vi "subExportDependencyItemRuleContent.vi"(8 "error in (no error)":errorcluster, 9 "Expand?":bool, 11 "IDependencyItemRule in":refnum<class "IDependencyItemRule.lvclass">) -> (0 "error out":errorcluster, 1 "Links":T1, 2 "Nodes":T1, 3 "IDependencyItemRule out":refnum<class "IDependencyItemRule.lvclass">)   [LabVIEW 2020, in "DefaultExtensions.lvlib" / "CGrapherDGML.lvclass"]
uses:
  CGrapherDGML.lvclass
  obj/Addons/LabVIEWObjectInterfaces.lvlibp/LabVIEWObjectInterfaces/IDependencyItemRule/IDependencyItemRule.lvclass
  C:/DependencyInspector/obj/Addons/LabVIEWObjectInterfaces.lvlibp/LabVIEWObjectInterfaces/ILabVIEWItem/ILabVIEWItem.lvclass
  obj/Addons/LabVIEWItem.lvlibp/LabVIEWItem/CLabVIEWItem/ConnectionSet.ctl
  84b6f64b-e02b-4565-8a95-97306d3fff3e.vi
  5ae37459-432d-44eb-8d2b-a2ae9b2d80af.vi
  0dec89c7-531e-457a-9eb0-0c91c63ee5dd.vi
  obj/Addons/LabVIEWItem.lvlibp/LabVIEWItem/CLabVIEWItem/CLabVIEWItem.lvclass
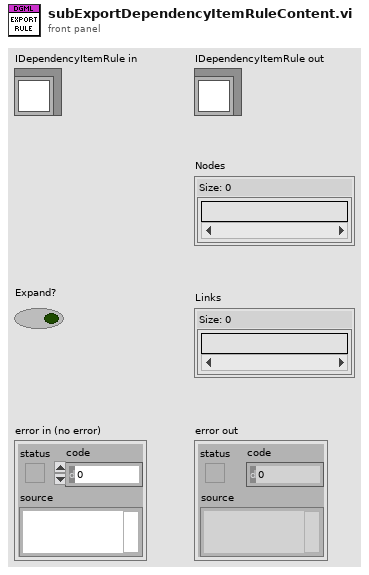
[diagram p1: front panel]
types:
  T1 = typedef "LabVIEWItem.lvlibp/CLabVIEWItem.lvclass/ConnectionSet.ctl" = set{string}
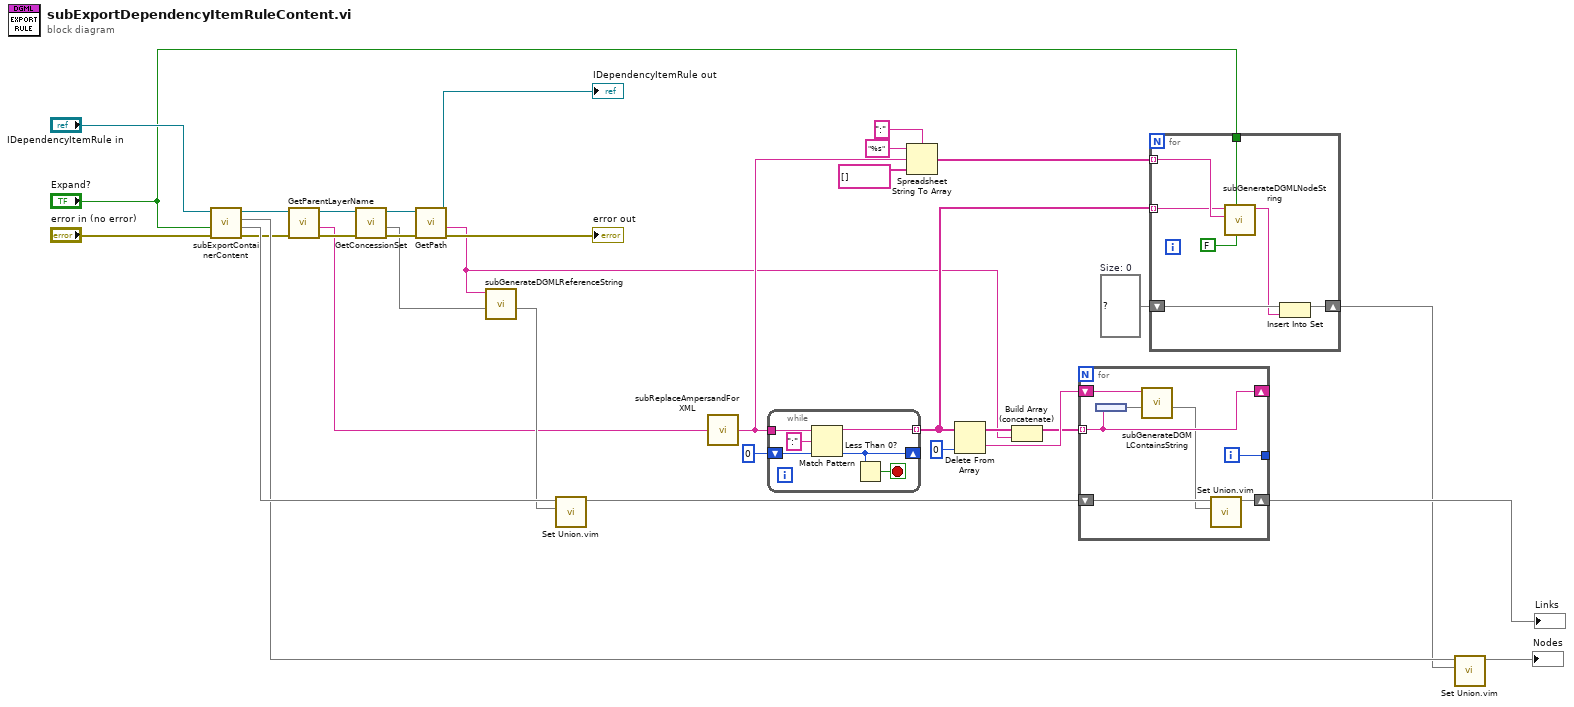
[diagram p0: block diagram]
diagram:
  w19 = set{string} {}  # Size: 0
  n1 = call "subExportContainerContent.vi"("error in (no error)"="error in (no error)", "Expand?"="Expand?", "ILabVIEWItem in"="IDependencyItemRule in") -> ("error out"=w4:errorcluster, "Links"=w30:T1, "Nodes"=w18:T1, "ILabVIEWItem out"=w5:refnum<class "IDependencyItemRule.lvclass">)  [unwired: 5 in]
  n2 = call-dynamic "GetParentLayerName.vi"("error in (no error)"=w4, "IDependencyItemRule in"=w5) -> ("error out"=w2:errorcluster, "Parent layer name"=w1:string, "IDependencyItemRule out"=w3:refnum<class "IDependencyItemRule.lvclass">)  [unwired: 7 in]
  n3 = call-dynamic "GetConcessionSet.vi"("error in (no error)"=w2, "IDependencyItemRule in"=w3) -> ("error out"=w7:errorcluster, "Concessions"=w6:set{string}, "IDependencyItemRule out"=w8:refnum<class "IDependencyItemRule.lvclass">)  [unwired: 7 in]
  n4 = call-dynamic "GetPath.vi"("error in (no error)"=w7, "ILabVIEWItem in"=w8) -> ("error out"=→"error out":errorcluster, "Path"=w10:string, "ILabVIEWItem out"=→"IDependencyItemRule out":refnum<class "IDependencyItemRule.lvclass">)  [unwired: 7 in]
  n5 = call "subGenerateDGMLReferenceString.vi"("References"=w6, "Source"=w10) -> ("Links"=w26:T1)  [unwired: 9 in]
  n6 = call "Set Union.vim"("set 2"=w26, "set 1"=w30) -> ("union"=w25:T1)  [unwired: 9 in]
  n7 = call "subReplaceAmpersandForXML.vi"("String"=w1) -> ("result string"=w24:string)
  n8 = while {
    tunnel: w24 -> [w39]
    shift-right: [w37] -> _
    shift-left: 0 ("offset past match") -> [w36]
    tunnel: [w34] -> w13 mode=indexing
    stop <- w35 stop-if-true
    n9 = Match Pattern(string=w39, regular expression=":" ("delimiter (Tab)"), offset (0)=w36) -> (before substring=w34:string, offset past match=w37:i32)  [unwired: 2 out]
    n10 = Less Than 0?(x=w37) -> (x < 0?=w35:bool)
  }
  n11 = Spreadsheet String To Array(delimiter (Tab)=":", format string="%s", spreadsheet string=w24, array type (2D Dbl)=string[] []) -> (array=w14:string[])
  n12 = Delete From Array(array=w13, index=0) -> (deleted portion=w27:string, array with subset deleted=w12:string[])  [unwired: 1 in]
  n13 = Build Array (concatenate)(w12, w10) -> (w11:string[])
  n14 = for {
    shift-right: [w44] -> _
    shift-left: w27 -> [w45]
    tunnel: w11 -> [w44] mode=indexing
    shift-right: [w40] -> w20
    shift-left: w25 -> [w42]
    tunnel: [w46] -> _
    i -> [w46]
    n15 = node(w44) -> (w43:set{string})
    n16 = call "subGenerateDGMLContainsString.vi"("Contained"=w43, "Source"=w45) -> ("Links"=w41:T1)  [unwired: 9 in]
    n17 = call "Set Union.vim"("set 2"=w41, "set 1"=w42) -> ("union"=w40:T1)  [unwired: 9 in]
  }
  "Links" <- w20
  n18 = for {
    tunnel: w14 -> [w53] mode=indexing
    tunnel: w13 -> [w52] mode=indexing
    shift-right: [w50] -> w16
    shift-left: w19 -> [w51]
    tunnel: "Expand?" -> [w47]
    n19 = call "subGenerateDGMLNodeString.vi"("Container empty?"=FALSE, "Expand?"=w47, "Label"=w53, "Id"=w52) -> ("Node string"=w49:string)  [unwired: 7 in]
    n20 = Insert Into Set(10:w49, 11:w51) -> (3:w50:set{string})  [unwired: 1 out]
  }
  n21 = call "Set Union.vim"("set 2"=w16, "set 1"=w18) -> ("union"=→"Nodes":T1)  [unwired: 9 in]
